vi "Time (SubVI).vi"(6 "Period":i64, 9 "Sim_Time [s]":dbl=82.0, 10 "stop RT":bool, 11 "Run_SIMULATION":bool) -> (1 "Stop":bool, 2 "SIM_Running":bool, 3 "i, sim_running, t[s], dt[s]":T1, 4 "Sim t [s]":dbl)   [LabVIEW 2017]
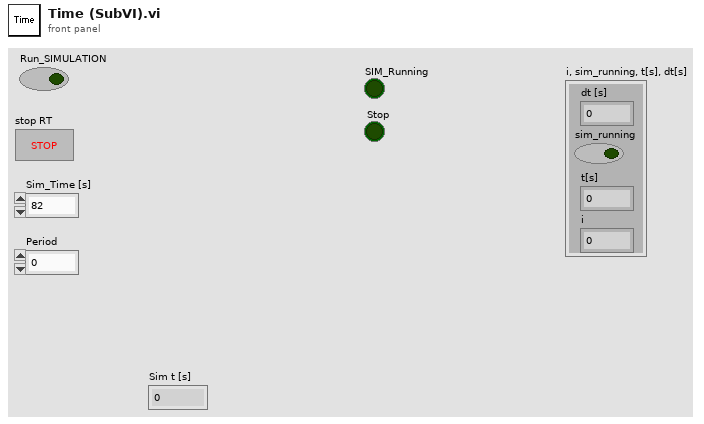
[diagram p1: front panel]
types:
  T1 = cluster{"dt [s]":dbl, "sim_running":bool, "t[s]":dbl, "i":i32}
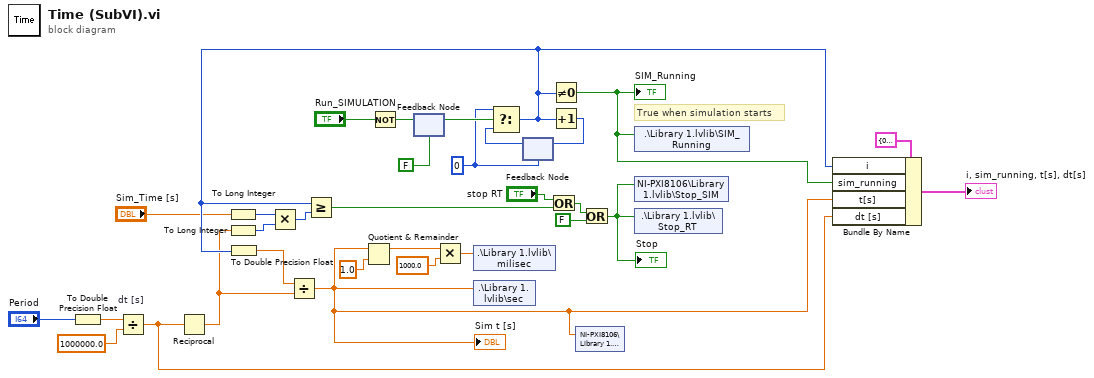
[diagram p0: block diagram]
diagram:
  w12 = 0 ("x")
  # "True when simulation starts"
  n1 = To Double Precision Float(number="Period") -> (double precision float=w4:dbl)
  n2 = Divide "dt [s]"(x=w4, y=1000000.0) -> (x/y=w28:dbl)
  n3 = Reciprocal(x=w28) -> (1/x=w7:dbl)
  n4 = To Long Integer(number="Sim_Time [s]") -> (32bit integer=w9:i32)
  n5 = To Long Integer(number=w7) -> (32bit integer=w6:i32)
  n6 = Multiply(x=w9, y=w6) -> (x*y=w2:i32)
  n7 = Not(x="Run_SIMULATION") -> (.not. x?=w18:bool)
  n8 = feedback #1(FALSE) -> (w22:bool)
  n9 = feedback-in #1(w18) -> ()
  n10 = feedback #2(w12) -> (w13:i32)
  n11 = Select(t=w12, s=w22, f=w13) -> (s? t:f=w27:i32)
  n12 = To Double Precision Float(number=w27) -> (double precision float=w8:dbl)
  n13 = Divide(x=w8, y=w7) -> (x/y=w1:dbl)
  "Sim t [s]" <- w1
  n14 = Greater Or Equal?(x=w27, y=w2) -> (x >= y?=w17:bool)
  n15 = Quotient & Remainder(x=w1, y=1.0) -> (x-y*floor(x/y)=w20:dbl)  [unwired: 1 out]
  n16 = Multiply(x=w20, y=1000.0) -> (x*y=w23:dbl)
  n17 = shared-variable ".\\Library 1.lvlib\\milisec"(w23) -> ()  [unwired: 1 in, 1 out]
  n18 = shared-variable ".\\Library 1.lvlib\\sec"(w1) -> ()  [unwired: 1 in, 1 out]
  n19 = Or(x="stop RT", y=w17) -> (x .or. y?=w24:bool)
  n20 = Not Equal To 0?(x=w27) -> (x != 0?=w26:bool)
  "SIM_Running" <- w26
  n21 = Increment(x=w27) -> (x+1=w11:i32)
  n22 = feedback-in #2(w11) -> ()
  n23 = shared-variable "NI-PXI8106\\Library 1.lvlib\\t"(w1) -> ()  [unwired: 1 in, 1 out]
  n24 = Or(x=w24, y=FALSE) -> (x .or. y?=w25:bool)
  "Stop" <- w25
  n25 = shared-variable ".\\Library 1.lvlib\\SIM_Running"(w26) -> ()  [unwired: 1 in, 1 out]
  n26 = shared-variable "NI-PXI8106\\Library 1.lvlib\\Stop_SIM"(w25) -> ()  [unwired: 1 in, 1 out]
  n27 = shared-variable ".\\Library 1.lvlib\\Stop_RT"(w25) -> ()  [unwired: 1 in, 1 out]
  n28 = Bundle By Name ("importante para o inicio")(cluster=T1 {"dt [s]"=0.0, "sim_running"=FALSE, "t[s]"=0.0, "i"=0} ("output cluster 2"), "i"=w27, "sim_running"=w26, "t[s]"=w1, "dt [s]"=w28) -> (→"i, sim_running, t[s], dt[s]":T1)
